vi "FW xy graph.vi"(0 "xy graph":cluster{"all rows":dbl[], "all rows":dbl[]}(graph), 1 "0.5 means FWHM":dbl=0.5 format="%.2f", 2 "length for BG subtraction (0=none)":i32) -> (3 "FWHM":dbl format="%.2f", 4 "max index(es)":i32, 5 "initial guess":T2={"initial amplitude"=nan, "initial center"=nan, "initial standard deviation"=nan, "offset"=nan}, 6 "FWHM pix":dbl format="%.2f")   [LabVIEW 2020]
uses:
  xy graph/interpolate xy graph options.ctl
  <vilib>/Analysis/baseanly.llb/Mean (DBL).vi
  <vilib>/Analysis/NI_AALBase.lvlib
panel:
  out "center x 2":dbl
  in  "Interpolate":cluster{"interp":bool, "interp options":T1}={"interp"=TRUE, "interp options"={"# samples (0=auto)"=10000, "auto maxmin"=TRUE, "x"={"max"=0.0, "min"=0.0}, "method"=2, "X is monotonic"=FALSE}} {"interp options"."method" items=["nearest", "linear", "spline", "cubic Hermite", "Lagrange"]}
  out "raw+interpolated":cluster{"xi used":dbl[], "yi":dbl[]}[](graph)
  out "half max rhs pix":dbl
  out "half max lhs pix":dbl
  out "peak y value":dbl
  out "center x value":dbl
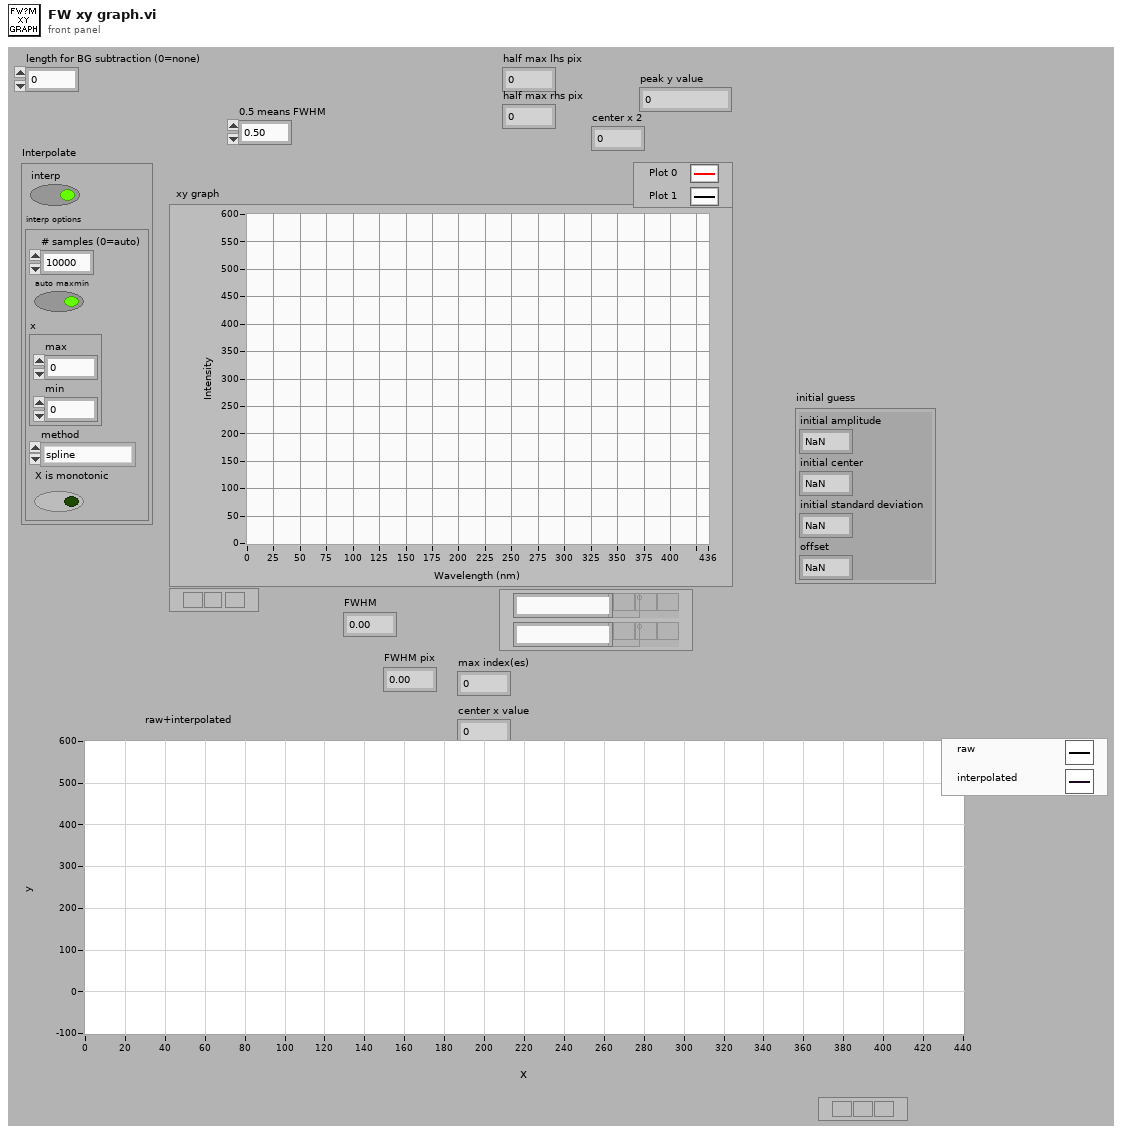
[diagram p1: front panel]
types:
  T1 = typedef "interpolate xy graph options.ctl" = cluster{"# samples (0=auto)":i32, "auto maxmin":bool, "x":cluster{"max":dbl, "min":dbl}, "method":i32, "X is monotonic":bool}
  T2 = cluster{"initial amplitude":dbl, "initial center":dbl, "initial standard deviation":dbl, "offset":dbl}
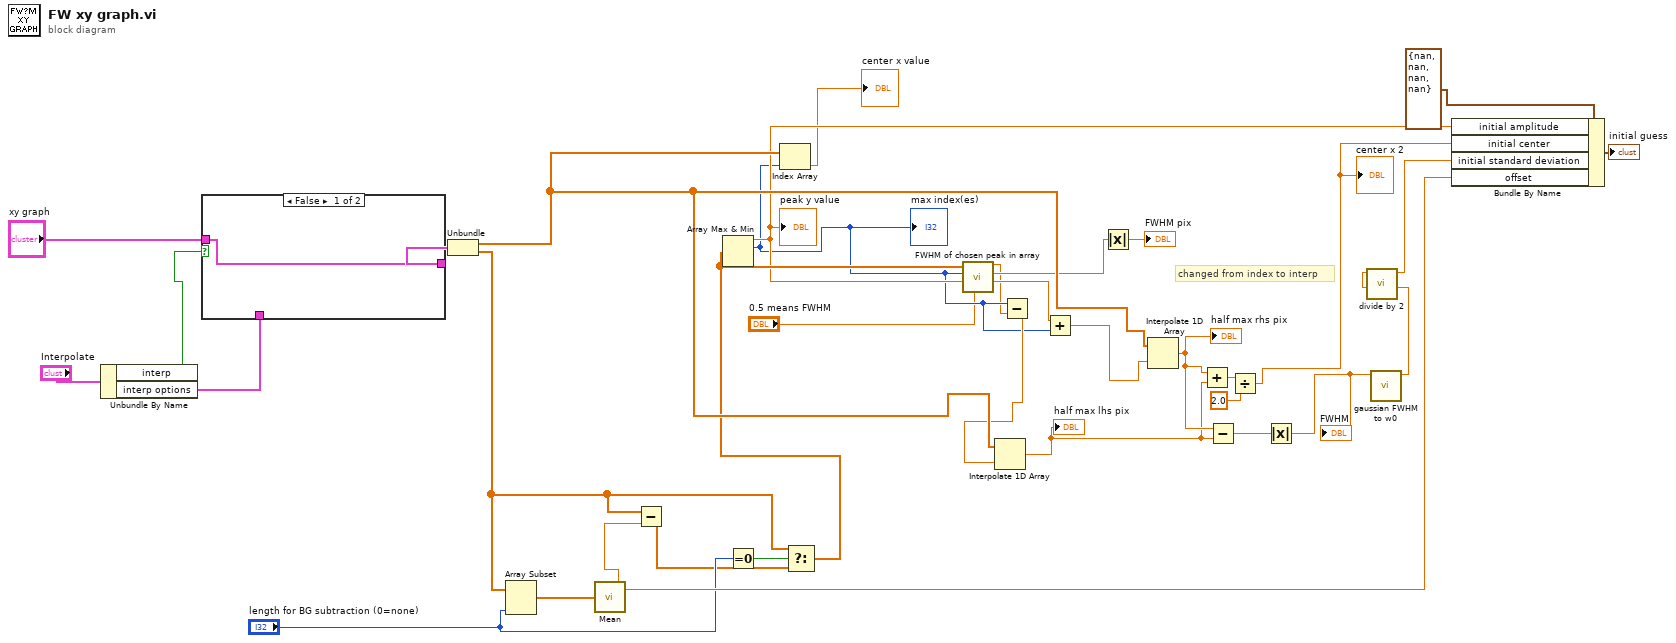
[diagram p0: block diagram]
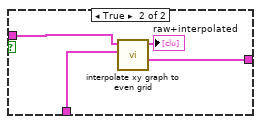
[diagram p2: hidden frame]
diagram:
  # "changed from index to interp"
  n1 = Unbundle By Name("Interpolate") -> ("interp"=w10:bool, "interp options"=w9:T1)
  n2 = case shown="False" w10 {
    tunnel: "xy graph" -> [w35 w39]
    tunnel: [w35 w38] -> w14
    tunnel: w9 -> [_ w36]
    frame False {
    }
    frame True {
      n3 = call "interpolate xy graph to even grid.vi"("interp options"=w36, "raw"=w39) -> ("interpolated"=w38:cluster{"xi used":dbl[], "yi":dbl[]}, "raw+interpolated"=→"raw+interpolated":cluster{"xi used":dbl[], "yi":dbl[]}[])  [unwired: 5 in, 3 out]
    }
  }
  n4 = Unbundle(w14) -> ("xi used"=w29:dbl[], "yi"=w17:dbl[])
  n5 = Array Subset(array=w17, length="length for BG subtraction (0=none)") -> (w31:dbl[])  [unwired: 1 in]
  n6 = call-poly <vilib>:"Mean.vi"("X"=w31) -> ("mean"=w28:dbl)  [unwired: 1 out]
  n7 = Subtract(x=w17, y=w28) -> (x-y=w25:dbl[])
  n8 = Equal To 0?(x="length for BG subtraction (0=none)") -> (x = 0?=w26:bool)
  n9 = Select(t=w17, s=w26, f=w25) -> (s? t:f=w24:dbl[])
  n10 = Array Max & Min(array=w24) -> (max value=w23:dbl, max index (indices)=w21:i32)  [unwired: 2 out]
  "max index(es)" <- w21
  "peak y value" <- w23
  n11 = Index Array(array=w29, index=w21) -> (element=→"center x value":dbl)
  n12 = call "FWHM of chosen peak in array.vi"("0.5 means FWHM"="0.5 means FWHM", "amplitude of peak"=w23, "index of peak"=w21, "counts"=w24) -> ("width of peak higher side"=w8:dbl, "FWHM"=w19:dbl, "width peak lower side"=w7:dbl)  [unwired: 5 in]
  n13 = Subtract(x=w21, y=w7) -> (x-y=w22:dbl)
  n14 = Interpolate 1D Array(1:w22, 2:w29) -> (0:w4:dbl)
  "half max lhs pix" <- w4
  n15 = Add(x=w8, y=w21) -> (x+y=w20:dbl)
  n16 = Absolute Value(x=w19) -> (abs(x)=→"FWHM pix":dbl)
  n17 = Interpolate 1D Array(1:w20, 2:w29) -> (0:w5:dbl)
  "half max rhs pix" <- w5
  n18 = Add(x=w5, y=w4) -> (x+y=w3:dbl)
  n19 = Subtract(x=w5, y=w4) -> (x-y=w32:dbl)
  n20 = Divide(x=w3, y=2.0) -> (x/y=w1:dbl)
  "center x 2" <- w1
  n21 = Absolute Value(x=w32) -> (abs(x)=w13:dbl)
  "FWHM" <- w13
  n22 = call "gaussian FWHM to w0.vi"("FWHM"=w13) -> ("w0"=w12:dbl)  [unwired: 10 in]
  n23 = call "divide by 2.vi"("Numeric in"=w12) -> ("Numeric out"=w16:dbl)  [unwired: 10 in]
  n24 = Bundle By Name(cluster=T2 {"initial amplitude"=nan, "initial center"=nan, "initial standard deviation"=nan, "offset"=nan} ("initial guess"), "initial amplitude"=w23, "initial center"=w1, "initial standard deviation"=w16, "offset"=w28) -> (→"initial guess":T2)
